vi "SiosIfmOpenCOM.vi"() -> ()   [LabVIEW 2009]
uses:
  siosifm.dll
panel:
  out "devNumber":i32
  in  "comNumber":i32
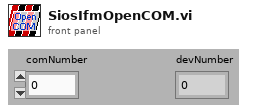
[diagram p1: front panel]
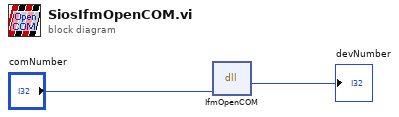
[diagram p0: block diagram]
diagram:
  n1 = dll-call lib="C:/WORK/Artem/RE-10/SIOS_IfmDLL/siosifm.dll" fn="IfmOpenCOM"("comNumber"="comNumber") -> ("devNumber"=→"devNumber":i32)  [unwired: 4 in, 2 out]
